vi "Display Select (SubVI).vi"(0 "CtlRef (Event)":refnum<vi>, 5 "Tab Ref":refnum<vi>, 9 "Config Ref":refnum<vi>, 11 "Help Ref":refnum<vi>, 12 "A Ref":refnum<vi>, 13 "B Ref":refnum<vi>, 14 "C Ref":refnum<vi>) -> ()   [LabVIEW 2010]
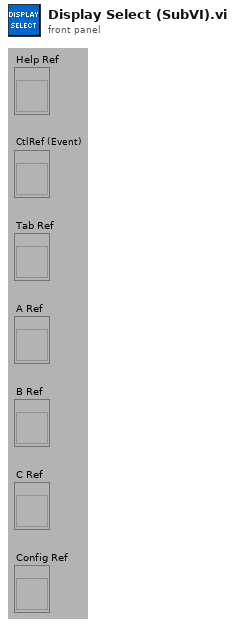
[diagram p1: front panel]
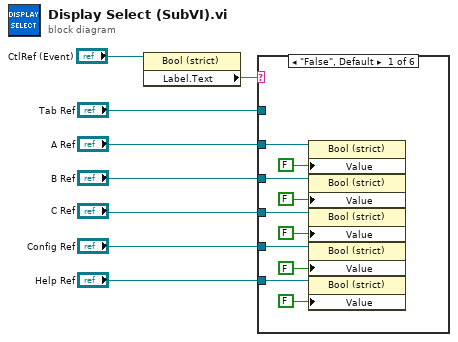
[diagram p0: block diagram]
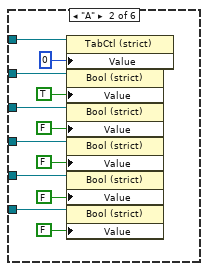
[diagram p2: hidden frame]
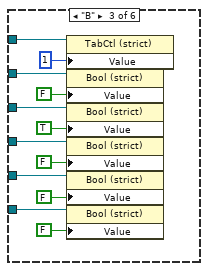
[diagram p3: hidden frame]
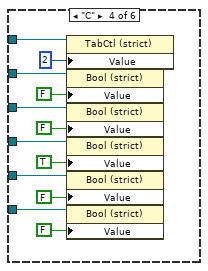
[diagram p4: hidden frame]
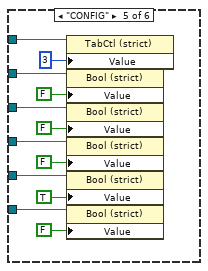
[diagram p5: hidden frame]
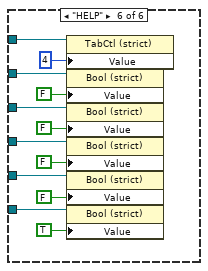
[diagram p6: hidden frame]
diagram:
  n1 = property class="Bool (strict)"(reference="CtlRef (Event)") -> ("Label.Text"=w8:string)  [unwired: 1 in, 2 out]
  n2 = case shown="\"False\", Default" w8 {
    tunnel: "Tab Ref" -> [_ w30 w42 w54 w66 w78]
    tunnel: "A Ref" -> [w13 w28 w40 w52 w64 w76]
    tunnel: "B Ref" -> [w12 w23 w35 w47 w59 w71]
    tunnel: "C Ref" -> [w11 w22 w34 w46 w58 w70]
    tunnel: "Config Ref" -> [w10 w21 w33 w45 w57 w69]
    tunnel: "Help Ref" -> [w9 w20 w32 w44 w56 w68]
    frame "False", Default {
      n3 = property class="Bool (strict)"(reference=w13, "Value"=FALSE) -> ()  [unwired: 1 in, 2 out]
      n4 = property class="Bool (strict)"(reference=w12, "Value"=FALSE) -> ()  [unwired: 1 in, 2 out]
      n5 = property class="Bool (strict)"(reference=w11, "Value"=FALSE) -> ()  [unwired: 1 in, 2 out]
      n6 = property class="Bool (strict)"(reference=w10, "Value"=FALSE) -> ()  [unwired: 1 in, 2 out]
      n7 = property class="Bool (strict)"(reference=w9, "Value"=FALSE) -> ()  [unwired: 1 in, 2 out]
    }
    frame "A" {
      n8 = property class="TabCtl (strict)"(reference=w30, "Value"=u32 0) -> ()  [unwired: 1 in, 2 out]
      n9 = property class="Bool (strict)"(reference=w28, "Value"=TRUE) -> ()  [unwired: 1 in, 2 out]
      n10 = property class="Bool (strict)"(reference=w23, "Value"=FALSE) -> ()  [unwired: 1 in, 2 out]
      n11 = property class="Bool (strict)"(reference=w22, "Value"=FALSE) -> ()  [unwired: 1 in, 2 out]
      n12 = property class="Bool (strict)"(reference=w21, "Value"=FALSE) -> ()  [unwired: 1 in, 2 out]
      n13 = property class="Bool (strict)"(reference=w20, "Value"=FALSE) -> ()  [unwired: 1 in, 2 out]
    }
    frame "B" {
      n14 = property class="TabCtl (strict)"(reference=w42, "Value"=u32 1) -> ()  [unwired: 1 in, 2 out]
      n15 = property class="Bool (strict)"(reference=w40, "Value"=FALSE) -> ()  [unwired: 1 in, 2 out]
      n16 = property class="Bool (strict)"(reference=w35, "Value"=TRUE) -> ()  [unwired: 1 in, 2 out]
      n17 = property class="Bool (strict)"(reference=w34, "Value"=FALSE) -> ()  [unwired: 1 in, 2 out]
      n18 = property class="Bool (strict)"(reference=w33, "Value"=FALSE) -> ()  [unwired: 1 in, 2 out]
      n19 = property class="Bool (strict)"(reference=w32, "Value"=FALSE) -> ()  [unwired: 1 in, 2 out]
    }
    frame "C" {
      n20 = property class="TabCtl (strict)"(reference=w54, "Value"=u32 2) -> ()  [unwired: 1 in, 2 out]
      n21 = property class="Bool (strict)"(reference=w52, "Value"=FALSE) -> ()  [unwired: 1 in, 2 out]
      n22 = property class="Bool (strict)"(reference=w47, "Value"=FALSE) -> ()  [unwired: 1 in, 2 out]
      n23 = property class="Bool (strict)"(reference=w46, "Value"=TRUE) -> ()  [unwired: 1 in, 2 out]
      n24 = property class="Bool (strict)"(reference=w45, "Value"=FALSE) -> ()  [unwired: 1 in, 2 out]
      n25 = property class="Bool (strict)"(reference=w44, "Value"=FALSE) -> ()  [unwired: 1 in, 2 out]
    }
    frame "CONFIG" {
      n26 = property class="TabCtl (strict)"(reference=w66, "Value"=u32 3) -> ()  [unwired: 1 in, 2 out]
      n27 = property class="Bool (strict)"(reference=w64, "Value"=FALSE) -> ()  [unwired: 1 in, 2 out]
      n28 = property class="Bool (strict)"(reference=w59, "Value"=FALSE) -> ()  [unwired: 1 in, 2 out]
      n29 = property class="Bool (strict)"(reference=w58, "Value"=FALSE) -> ()  [unwired: 1 in, 2 out]
      n30 = property class="Bool (strict)"(reference=w57, "Value"=TRUE) -> ()  [unwired: 1 in, 2 out]
      n31 = property class="Bool (strict)"(reference=w56, "Value"=FALSE) -> ()  [unwired: 1 in, 2 out]
    }
    frame "HELP" {
      n32 = property class="TabCtl (strict)"(reference=w78, "Value"=u32 4) -> ()  [unwired: 1 in, 2 out]
      n33 = property class="Bool (strict)"(reference=w76, "Value"=FALSE) -> ()  [unwired: 1 in, 2 out]
      n34 = property class="Bool (strict)"(reference=w71, "Value"=FALSE) -> ()  [unwired: 1 in, 2 out]
      n35 = property class="Bool (strict)"(reference=w70, "Value"=FALSE) -> ()  [unwired: 1 in, 2 out]
      n36 = property class="Bool (strict)"(reference=w69, "Value"=FALSE) -> ()  [unwired: 1 in, 2 out]
      n37 = property class="Bool (strict)"(reference=w68, "Value"=TRUE) -> ()  [unwired: 1 in, 2 out]
    }
  }
